vi "Pane Resize.vi"(6 "Control Ref Queue":T1, 8 "error in (no error)":errorcluster) -> (0 "error out":errorcluster)   [LabVIEW 2017, in "XY Plot Matrix.lvclass"]
uses:
  <vilib>/Math Plots/2D Math Plots/XY Plot Matrix/XY Plot Matrix/XY Plot Matrix.lvclass
  <vilib>/Math Plots/2D Math Plots/2D Plot/Action String/XYPlotMatrix Ctrl Act Queue.ctl
  <vilib>/Math Plots/2D Math Plots/2D Plot/Action String/XYPlotMatrix Ctrl Act Cluster.ctl
  <vilib>/Math Plots/2D Math Plots/2D Plot/Action String/2DMathPlot State Class.ctl
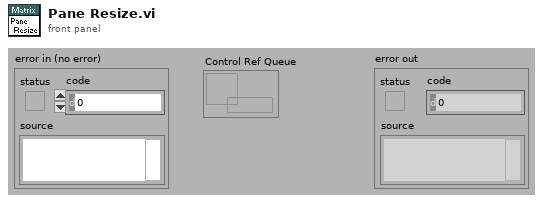
[diagram p1: front panel]
types:
  T1 = typedef "XYPlotMatrix Ctrl Act Queue.ctl" = refnum<queue>
  T2 = typedef "XYPlotMatrix Ctrl Act Cluster.ctl" = cluster{"Facade VI":refnum<vi>, "XControl":refnum<vi>, "Sub Panel":refnum<vi>, "Sub VI":refnum<vi>, "Export Image":refnum<vi>, "Display State Change Class":T3}
  T3 = typedef "2DMathPlot State Class.ctl" = enum16{"Update All (Undo)", "Update General", "Update Appearance", "Update Format", "Update Scale", "Update Marker", "Update Cursor", "None"}
  T4 = typedef "LVBoundsTypeDef.ctl" = cluster{"Width":u32, "Height":u32}
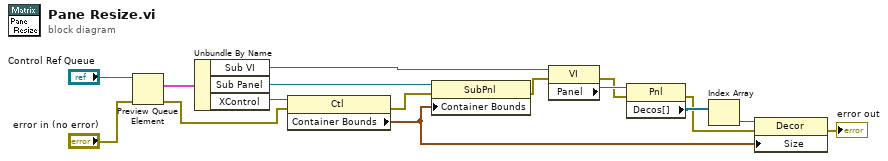
[diagram p0: block diagram]
diagram:
  n1 = Preview Queue Element(queue="Control Ref Queue", error in (no error)="error in (no error)") -> (element=w14:T2, error out=w11:errorcluster)  [unwired: 3 out]
  n2 = Unbundle By Name(w14) -> ("Sub VI"=w9:refnum<vi>, "Sub Panel"=w12:refnum<vi>, "XControl"=w13:refnum<vi>)
  n3 = property class="Ctl"(reference=w13, error in=w11) -> (error out=w10:errorcluster, "Container Bounds"=w5:T4)  [unwired: 1 out]
  n4 = property class="SubPnl"(reference=w12, error in=w10, "Container Bounds"=w5) -> (error out=w3:errorcluster)  [unwired: 1 out]
  n5 = property class="VI"(reference=w9, error in=w3) -> (error out=w4:errorcluster, "Panel"=w8:refnum<vi>)  [unwired: 1 out]
  n6 = property class="Pnl"(reference=w8, error in=w4) -> (error out=w2:errorcluster, "Decos[]"=w7:refnum<vi>[])  [unwired: 1 out]
  n7 = Index Array(array=w7) -> (element=w6:refnum<vi>)  [unwired: 1 in]
  n8 = property class="Decor"(reference=w6, error in=w2, "Size"=w5) -> (error out=→"error out":errorcluster)  [unwired: 1 out]
